vi "Set Error.vi"(10 "Error":errorcluster, 11 "Self Actor in":refnum<class "Self Actor.lvclass">) -> (3 "Self Actor out":refnum<class "Self Actor.lvclass">)   [LabVIEW 2021, in "jettl.lvlib" / "Self Actor.lvclass"]
uses:
  Self Actor.lvclass
  Self Actor.lvclass/Self Actor.ctl
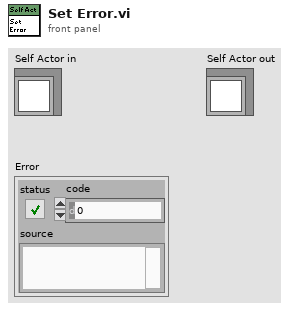
[diagram p1: front panel]
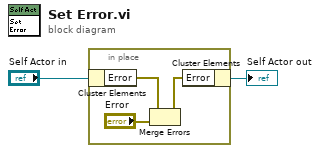
[diagram p0: block diagram]
diagram:
  n1 = in-place {
    n2 = in-place-cluster #1("Self Actor in") -> ("Error"=w5:errorcluster)
    n3 = Merge Errors(w5, "Error") -> (w4:errorcluster)
    n4 = in-place-cluster #1("Error"=w4) -> (→"Self Actor out":refnum<class "Self Actor.lvclass">)
  }
